vi "Check if Class is Test Case.vi"(8 "error in (no error)":errorcluster, 11 "Path":path) -> (0 "error out":errorcluster, 3 "Is Test Case?":bool)   [LabVIEW 2020, in "Utilities.lvlib"]
uses:
  Utilities.lvlib
  Test Case/LUnit Test Case.lvclass
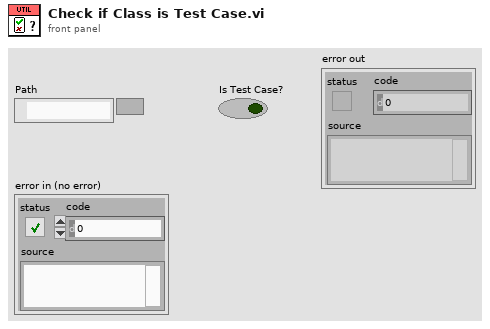
[diagram p1: front panel]
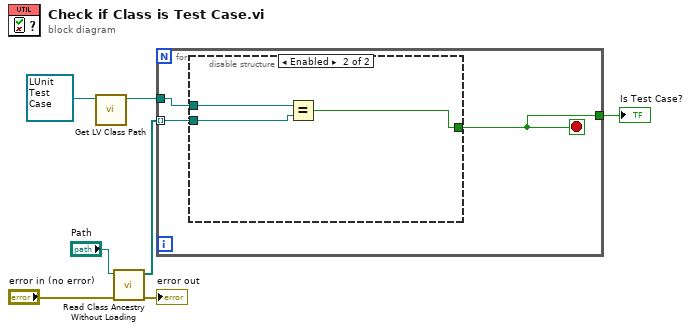
[diagram p0: block diagram]
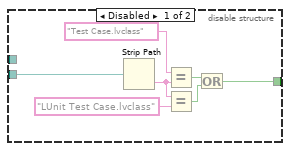
[diagram p2: hidden frame]
diagram:
  n1 = call <vilib>:"Get LV Class Path.vi"("object"=refnum<class "LUnit Test Case.lvclass"> refnum ("LUnit Test Case.lvclass")) -> ("class path"=w1:path)  [unwired: 9 in, 1 out]
  n2 = call <vilib>:"Read Class Ancestry Without Loading.vi"("error in (no error)"="error in (no error)", "LabVIEW Class Path"="Path") -> ("error out"=→"error out":errorcluster, "Class Ancestry"=w6:path[])  [unwired: 8 in]
  n3 = for {
    tunnel: [w9] -> w4
    tunnel: w6 -> [w10] mode=indexing
    tunnel: w1 -> [w8]
    stop <- w9 stop-if-true
    n4 = disable-structure shown="Enabled" {
      disable-tunnel: w10 -> [w16 w19]
      disable-tunnel: [w14 w18] -> w9
      disable-tunnel: w8 -> [_ w20]
      frame Disabled {
        n5 = Strip Path(path=w16) -> (name=w12:string)  [unwired: 1 out]
        n6 = Equal?(x="Test Case.lvclass" ("class path"), y=w12) -> (x = y?=w17:bool)
        n7 = Equal?(x=w12, y="LUnit Test Case.lvclass" ("class path")) -> (x = y?=w11:bool)
        n8 = Or(x=w17, y=w11) -> (x .or. y?=w14:bool)
      }
      frame Enabled {
        n9 = Equal?(x=w20, y=w19) -> (x = y?=w18:bool)
      }
    }
  }
  "Is Test Case?" <- w4
